vi "Class - Class Private Data.vi"(7 "Msg Chain":string, 8 "error in (no error)":errorcluster {"code" format="Error %.0f"}, 10 "Classes":refnum<class "Class Documentation.lvclass">[](array[class]), 11 "VIDoc Printer - Confluence In":refnum<class "VIDoc Printer - Confluence.lvclass">) -> (0 "error out":errorcluster {"code" format="Error %.0f"}, 3 "VIDoc Printer - Confluence Out":refnum<class "VIDoc Printer - Confluence.lvclass">)   [LabVIEW 2023, in "VIDoc Printer - Confluence.lvlib" / "VIDoc Printer - Confluence.lvclass"]
uses:
  VIDoc Printer - Confluence.lvclass
  C:/projects/DMC/Tooling/Git-Action-Service/Source/Documentation Generation/Printers/Printer/VIDoc Printer.lvclass
  Parsing/Class Documentation/Class Documentation.lvclass
  Parsing/Class Documentation/Class Documentation.lvclass/Class Documentation.ctl
  Printer/VIDoc Printer.lvclass/VIDoc Printer.ctl
  Confluence Formatting/Types/Format Combo Box.ctl
  VIDoc Printer - Confluence.lvclass/VIDoc Printer - Confluence.ctl
  Accessors/Get Class CPD Expand.vi
  Printer/Accessors/Get Class Settings - CPD Detail Level.vi
  Parsing/Class Documentation/Get Class Private Data.vi
  Parsing/Class Documentation/Get Name.vi
  Printer/VIDoc Printer.lvclass
  UI Interaction/UI Interaction.lvclass
  Confluence Formatting/Confluence Formatting.lvlib
  C:/projects/DMC/Tooling/Git-Action-Service/Source/Documentation Generation/Printers/Confluence Printer/VIDoc Printer - Confluence.lvclass
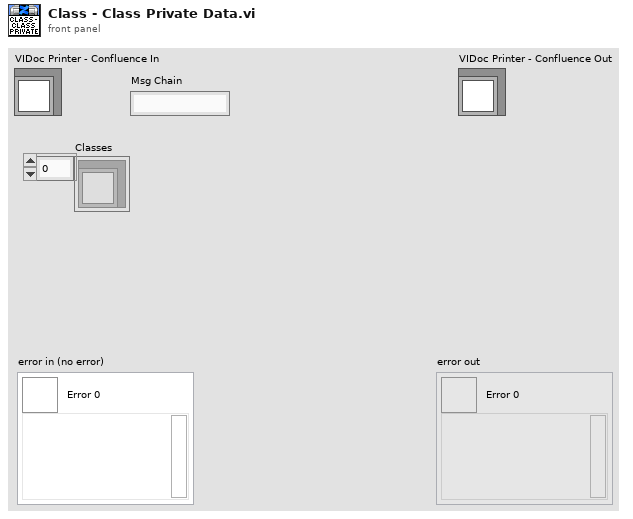
[diagram p1: front panel]
types:
  T1 = typedef "Confluence Formatting.lvlib/Format Combo Box.ctl" = string
  T2 = typedef "VIDoc Parsing.lvlib/Controls Info Cluster.ctl" = cluster{"Name":string, "Description":string, "Data Type":string, "Tip Strip":string, "UID":i32, "Image Data":T3, "ToggleKeyBind":T4, "Raw Label":string, "Raw Caption":string}
  T3 = typedef "imagedata.ctl" = cluster{"image type":i32, "image depth":i32, "image":u8[], "mask":u8[], "colors":u32[], "Rectangle":cluster{"left":i16, "top":i16, "right":i16, "bottom":i16}}
  T4 = typedef "LVKeyTypeDef.ctl" = cluster{"Focus":bool, "Control":bool, "Shift":bool, "Key":string}
  T5 = typedef "VIDoc Printer.lvlib/Printer Settings.lvclass/Detail Level Enum.ctl" = enum16{"None", "Minimal", "Standard", "Full"}
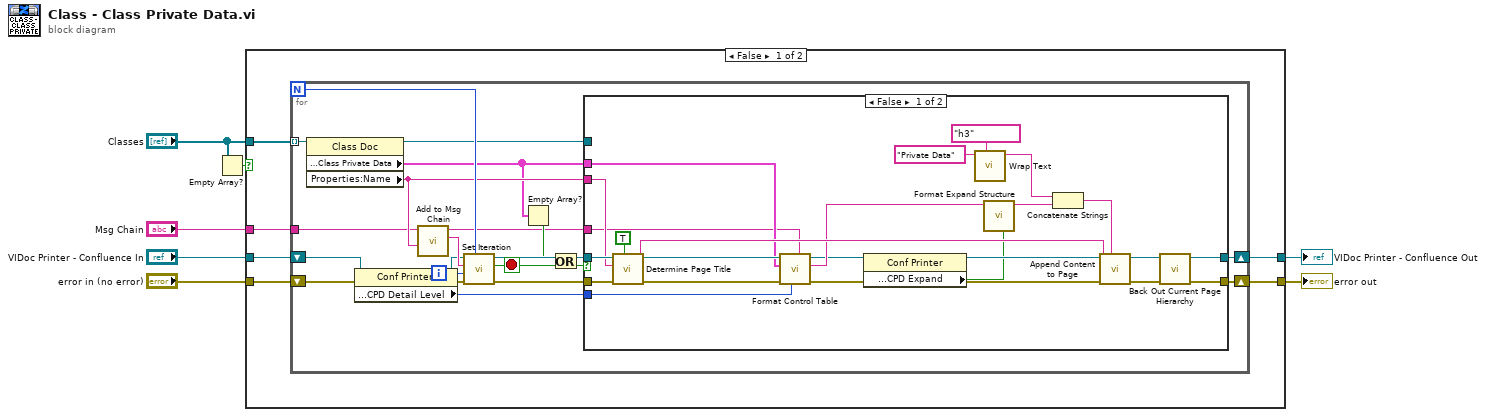
[diagram p0: block diagram]
diagram:
  n1 = Empty Array?(array="Classes") -> (empty?=w7:bool)
  n2 = case shown="False" w7 {
    tunnel: [w13 w60] -> w6
    tunnel: [w12 w61] -> w5
    tunnel: "error in (no error)" -> [w11 w60]
    tunnel: "Classes" -> [w10 _]
    tunnel: "VIDoc Printer - Confluence In" -> [w9 w61]
    tunnel: "Msg Chain" -> [w8 _]
    frame False {
      n3 = for {
        N -> [w27]
        shift-right: [w31] -> w13
        shift-left: w11 -> [w30]
        shift-right: [w32] -> w12
        shift-left: w9 -> [w20]
        tunnel: w10 -> [w33] mode=indexing
        tunnel: w8 -> [w14]
        i -> [w26]
        stop <- w23 stop-if-true
        n4 = property class="Class Doc"(reference=w33) -> (reference out=w22:refnum<class "Class Documentation.lvclass">, "Properties:Class Private Data"=w18:T2[], "Properties:Name"=w25:string)  [unwired: 1 in, 1 out]
        n5 = property class="Conf Printer"(reference=w20, error in=w30) -> (reference out=w19:refnum<class "VIDoc Printer - Confluence.lvclass">, error out=w21:errorcluster, "Properties:Settings:Classes:CPD Detail Level"=w15:T5)
        n6 = call "Add to Msg Chain.vi"("New"=w25, "Msg Chain in"=w14) -> ("Msg Chain out"=w24:string)  [unwired: 9 in]
        n7 = call "Set Iteration.vi"("Progress Max"=w27, "error in (no error)"=w21, "Progress Value"=w26, "Message (No Message Update)"=w24, "VIDoc Printer In"=w19) -> ("error out"=w28:errorcluster, "Abort?"=w23:bool, "VIDoc Printer Out"=w29:refnum<class "VIDoc Printer - Confluence.lvclass">)  [unwired: 4 in]
        n8 = Empty Array?(array=w18) -> (empty?=w16:bool)
        n9 = Or(x=w16, y=w23) -> (x .or. y?=w17:bool)
        n10 = case shown="False" w17 {
          tunnel: [w41 w58] -> w32
          tunnel: [w40 w59] -> w31
          tunnel: w18 -> [w45 _]
          tunnel: w29 -> [w55 w58]
          tunnel: w28 -> [w54 w59]
          tunnel: w25 -> [w53 _]
          tunnel: w22 -> [_ _]
          tunnel: w15 -> [w39 _]
          tunnel: w14 -> [w34 _]
          frame False {
            n11 = call "Determine Page Title.vi"("Update Current Page (F)"=TRUE, "error in (no error)"=w54, "Name"=w53, "VIDoc Printer - Confluence In"=w55) -> ("error out"=w48:errorcluster, "Page Title"=w57:string, "VIDoc Printer - Confluence Out"=w49:refnum<class "VIDoc Printer - Confluence.lvclass">)  [unwired: 4 in, 1 out]
            n12 = call "Format Control Table.vi"("Msg Chain in"=w34, "Controls Opt"=w39, "error in (no error)"=w48, "Controls"=w45, "VIDoc Printer - Confluence In"=w49) -> ("error out"=w47:errorcluster, "Table"=w46:string, "VIDoc Printer - Confluence Out"=w38:refnum<class "VIDoc Printer - Confluence.lvclass">)  [unwired: 4 in]
            n13 = property class="Conf Printer"(reference=w38) -> (reference out=w37:refnum<class "VIDoc Printer - Confluence.lvclass">, "Properties:Expand?:Class:CPD Expand"=w35:bool)  [unwired: 1 in, 1 out]
            n14 = call "Wrap Text.vi"("Formatting"=T1 "h3", "String"="Private Data") -> ("Wrapped String"=w51:string)  [unwired: 8 in, 1 out]
            n15 = call "Format Expand Structure.vi"("Enable? (T)"=w35, "Content"=w46) -> ("Expand String"=w36:string)  [unwired: 8 in, 1 out]
            n16 = Concatenate Strings(w51, w36) -> (w50:string)
            n17 = call "Append Content to Page.vi"("Page Content"=w50, "error in (no error)"=w47, "Page Title"=w57, "VIDoc Printer - Confluence In"=w37) -> ("error out"=w42:errorcluster, "VIDoc Printer - Confluence Out"=w43:refnum<class "VIDoc Printer - Confluence.lvclass">)  [unwired: 6 in]
            n18 = call "Back Out Current Page Hierarchy.vi"("error in (no error)"=w42, "VIDoc Printer - Confluence In"=w43) -> ("error out"=w40:errorcluster, "VIDoc Printer - Confluence Out"=w41:refnum<class "VIDoc Printer - Confluence.lvclass">)  [unwired: 8 in]
          }
          frame True {
          }
        }
      }
    }
    frame True {
    }
  }
  "error out" <- w6
  "VIDoc Printer - Confluence Out" <- w5
